vi "UDP+Command.vi"() -> ()   [LabVIEW 2019, in "Part of Main VIs.lvlib" / "Command Library.lvlib"]
uses:
  Command Library.lvlib
  <vilib>/Utility/error.llb/DialogType.ctl
  <extravilib>/ChannelInstances/Tag-str/Read With Abort.vi
  <extravilib>/ChannelInstances/Tag-str/Write With Abort.vi
  <extravilib>/ChannelInstances/Tag-str/Instantiate.vi
  <extravilib>/ChannelInstances/Tag-str/EndpointRead.vi
  <extravilib>/ChannelInstances/Tag-str/Endpoint.vi
  <extravilib>/ChannelInstances/Tag-str.lvlib
panel:
  in  "error in (no error)":errorcluster
  out "error out":errorcluster
  out "InterfaceName":string
  out "SlotNo":string
  out "ChannelNo":string
  out "Status":string
  out "Value":string
  out "Sender IP Adress for Command PC":string
  out "Datagram Port for Command PC":u16
  out "Listening Port for Command PC":u16
  out "Command Read?":bool
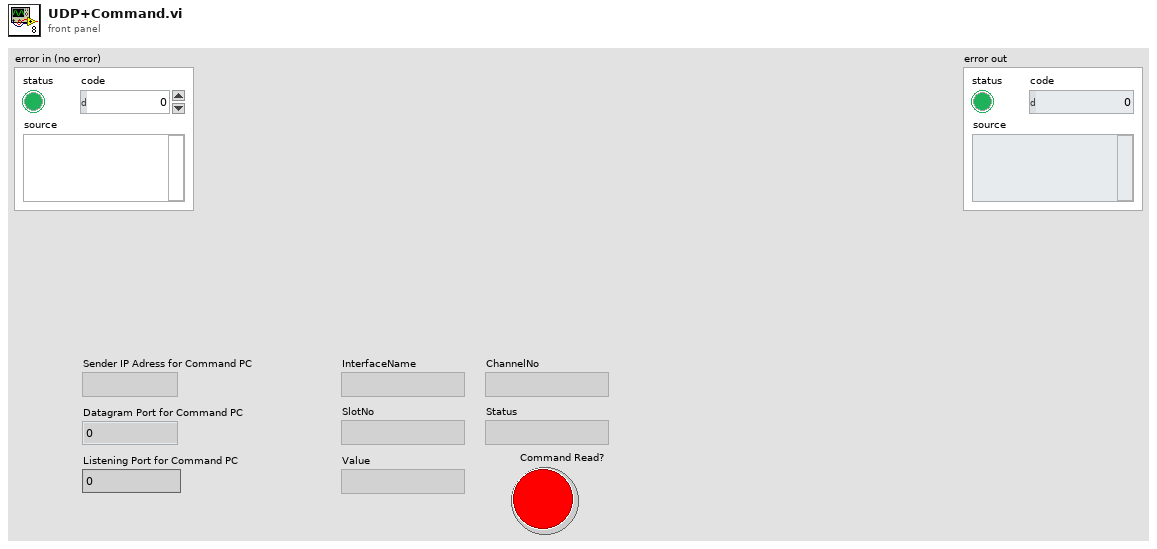
[diagram p1: front panel]
types:
  T1 = typedef "DialogType.ctl" = u16
  T2 = typedef "Tag-str.lvlib/))Channel.ctl" = refnum<queue>
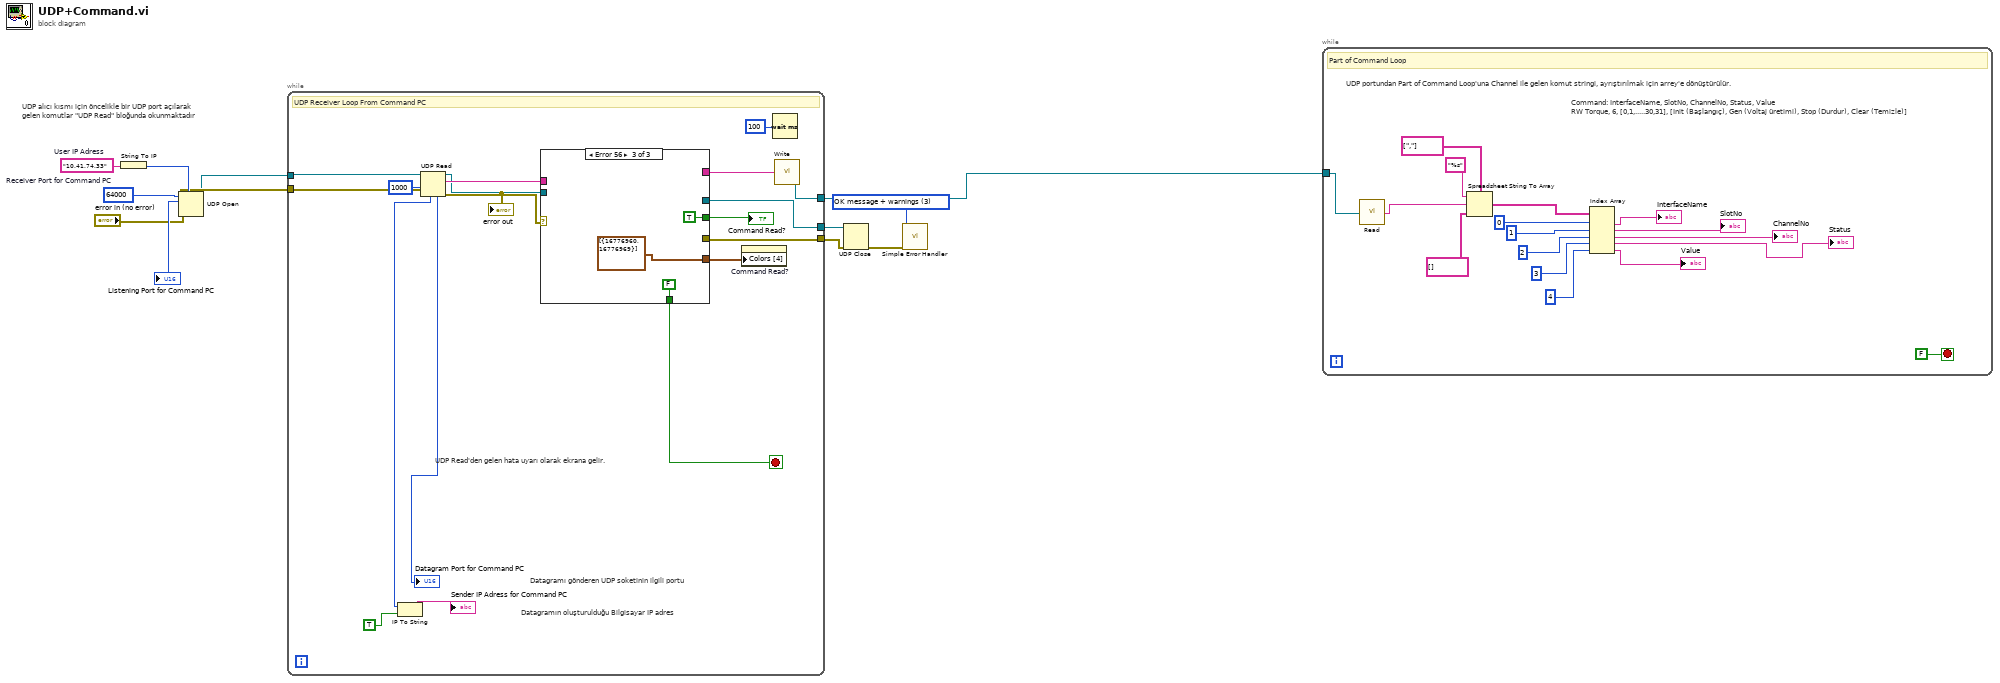
[diagram p0: block diagram]
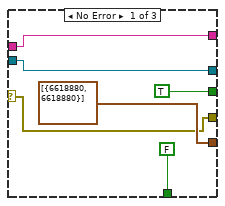
[diagram p2: hidden frame]
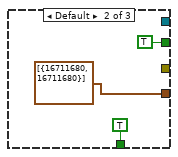
[diagram p3: hidden frame]
diagram:
  w4 = T1 3 items=["no dialog", "OK message", "continue or stop message", "OK message + warnings", "continue/stop + warnings"] ("type of dialog (OK msg:1)")
  w10 = u16 64000  # Receiver Port for Command PC
  w12 = "10.41.74.33"  # User IP Adress
  # "UDP alıcı kısmı için öncelikle bir UDP port açılarak \ngelen komutlar \"UDP Read\" bloğunda okunmaktadır"
  n1 = String To IP(1:w12) -> (0:w11:u32)
  n2 = UDP Open(7:w11, 8:"error in (no error)", 11:w10) -> (port=w8:refnum<k16>, 0:w9:errorcluster, 2:→"Listening Port for Command PC":u16)  [unwired: 2 in]
  n3 = while {
    tunnel: w9 -> [w30]
    tunnel: w8 -> [w21]
    tunnel: [w29] -> w5
    tunnel: [w16] -> w3
    tunnel: [w15] -> w2
    stop <- w20 stop-if-true
    # "Datagramın oluşturulduğu Bilgisayar IP adres"
    # "Datagramı gönderen UDP soketinin ilgili portu"
    # "UDP Read'den gelen hata uyarı olarak ekrana gelir."
    # "UDP Receiver Loop From Command PC"
    n4 = UDP Read(connection ID=w21, timeout ms (25000)=1000, 8:w30) -> (data out=w18:string, error out=w19:errorcluster, 3:w14:refnum<k16>, 4:→"Datagram Port for Command PC":u16, 6:w23:u32)  [unwired: 1 in]
    "error out" <- w19
    n5 = IP To String(1:TRUE ("dot notation? (F)"), 2:w23) -> (0:→"Sender IP Adress for Command PC":string)
    n6 = case shown="Error 56" w19 {
      selector: w19 -> [w32 _ _]
      tunnel: [TRUE ("UDP Read?") TRUE ("UDP Read?") TRUE ("UDP Read?")] -> w27
      tunnel: [cluster{u32, u32}[] [{6618880, 6618880}] ("Colors [4]") cluster{u32, u32}[] [{16711680, 16711680}] ("Colors [4]") cluster{u32, u32}[] [{16776960, 16776969}] ("Colors [4]")] -> w26
      tunnel: [FALSE TRUE FALSE] -> w20
      tunnel: w18 -> [w33 _ _]
      tunnel: [w33 _ _] -> w17
      tunnel: [w32 _ _] -> w16
      tunnel: [w31 _ _] -> w15
      tunnel: w14 -> [w31 _ _]
      frame No Error {
      }
      frame Default {
      }
      frame Error {
      }
    }
    "Command Read?" <- w27
    n7 = property on="Command Read?" class="Bool (strict)"("Colors [4]"=w26) -> ()  [unwired: 2 in, 2 out]
    n8 = Wait (ms)(milliseconds to wait=u32 100) -> ()  [unwired: 1 out]
    n9 = call <extravilib>:"Write.vi"("element"=w17) -> ("channel"=w29:T2)  [unwired: 1 out]
  }
  n10 = UDP Close(connection ID=w2, 8:w3) -> (error out=w7:errorcluster)  [unwired: 1 out]
  n11 = call <vilib>:"Simple Error Handler.vi"("type of dialog (OK msg:1)"=w4, "error in (no error)"=w7) -> ()  [unwired: 3 in, 5 out]
  n12 = while {
    tunnel: w5 -> [w44]
    stop <- FALSE stop-if-true
    # "UDP portundan Part of Command Loop'una Channel ile gelen komut stringi, ayrıştırılmak için arrey'e dönüştürülür."
    # "Command: InterfaceName, SlotNo, ChannelNo, Status, Value\nRW Torque, 6, [0,1,.....30,31], [Init (Başlangıç), Gen (Voltaj üretimi), Stop (Durdur), Clear (Temizle)]"
    # "Part of Command Loop"
    n13 = call <extravilib>:"Read.vi"("channel"=w44) -> ("element"=w52:string)  [unwired: 1 in, 1 out]
    n14 = Spreadsheet String To Array(delimiter (Tab)=string[] [","], format string="%s", spreadsheet string=w52, array type (2D Dbl)=string[] [] ("Array")) -> (array=w57:string[])
    n15 = Index Array "Index Array"(array=w57, index #1=0 ("index"), index #2=1 ("index"), index #3=2 ("index"), index #4=3 ("index"), index #5=4 ("index")) -> (element #1=→"InterfaceName":string, element #2=→"SlotNo":string, element #3=→"ChannelNo":string, element #4=→"Status":string, element #5=→"Value":string)
  }
